vi "PumpStop_all.vi"(8 "Error In":errorcluster, 11 "Pump COMM Port":refnum<visa-resource-name>) -> (0 "Error Out":errorcluster)   [LabVIEW 2015]
panel:
  in  "Pump Address":string[](array[string])=["e", "g", "h", "i", "j", "f"]
  # "Stop All Micro Lynx Milligat Pumps"
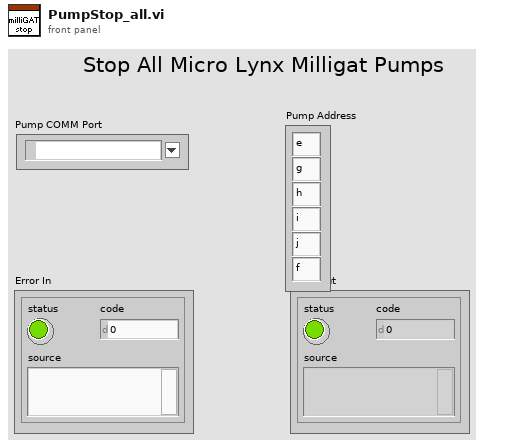
[diagram p1: front panel]
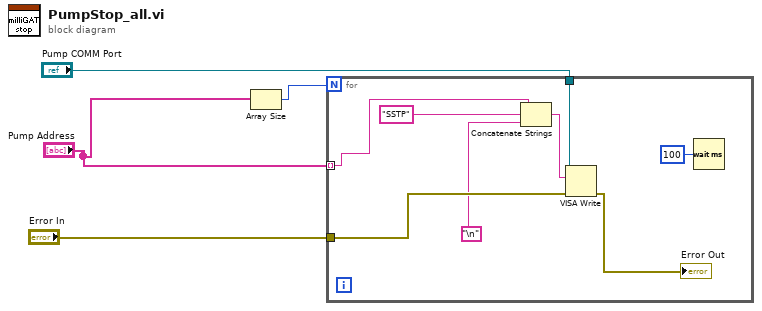
[diagram p0: block diagram]
diagram:
  n1 = Array Size(array="Pump Address") -> (size(s)=w2:i32)
  n2 = for {
    N: w2 -> [_]
    tunnel: "Error In" -> [w11]
    tunnel: "Pump COMM Port" -> [w8]
    tunnel: "Pump Address" -> [w6] mode=indexing
    n3 = Concatenate Strings(w6, "SSTP", "\n") -> (w12:string)
    n4 = VISA Write(VISA resource name=w8, write buffer=w12, error in (no error)=w11) -> (error out=→"Error Out":errorcluster)  [unwired: 2 out]
    n5 = Wait (ms)(milliseconds to wait=u32 100) -> ()  [unwired: 1 out]
  }
